vi "PC_AIChar.vi"() -> ()   [LabVIEW 2017]
uses:
  <vilib>/NI/STM/NI STM.lvlib
  <vilib>/Analysis/NI_AALBase.lvlib
  <vilib>/measure/NI_MAPro.lvlib
  <vilib>/measure/maspectr.llb/Power Spectrum and PSD Export Mode.ctl
  <vilib>/Analysis/NI_AALPro.lvlib
  Components/TypeDefs/UIStateDefEnum.ctl
  Components/Spectra/Spectra.lvlib
  <vilib>/NI/STM/TCP/Read Message (TCP).vi
  <vilib>/Analysis/5stat.llb/RMS (DBL).vi
  <vilib>/measure/maspectr.llb/FFT Power Spectrum and PSD for 1 Chan.vi
  <vilib>/Analysis/baseanly.llb/Mean (DBL).vi
  <vilib>/NI/STM/TCP/Read Meta Data (TCP Ref).vi
  <vilib>/NI/STM/TCP/Get Connection Reference (TCP).vi
panel:
  out "Analysis Loop \ntime [s]":dbl format="%#.4g"
  out "Analysis \ntime-span [s]":dbl format="%.2f"
  out "# of elements \nremoved":i32
  in  "Pause Charts":bool
  in  "Clear charts":bool
  out "RT target \nloop \ntime [s]":dbl=0.0002
  out "Data length \n[count]":i32
  out "Mean [V]":dbl format="%#.6f"
  out "RMS / \nStd. Dev. [mV]":dbl format="%#.6f"
  out "Spectra plots":cluster{"f0":dbl, "df":dbl, "magnitude":dbl[]}[](graph)
  out "Histogram Graph":T1(graph)
  out "STM Loop \ntime [s]":dbl format="%#.4g"
  in  "System Stop Button":bool
  out "Data":dbl[][](graph)
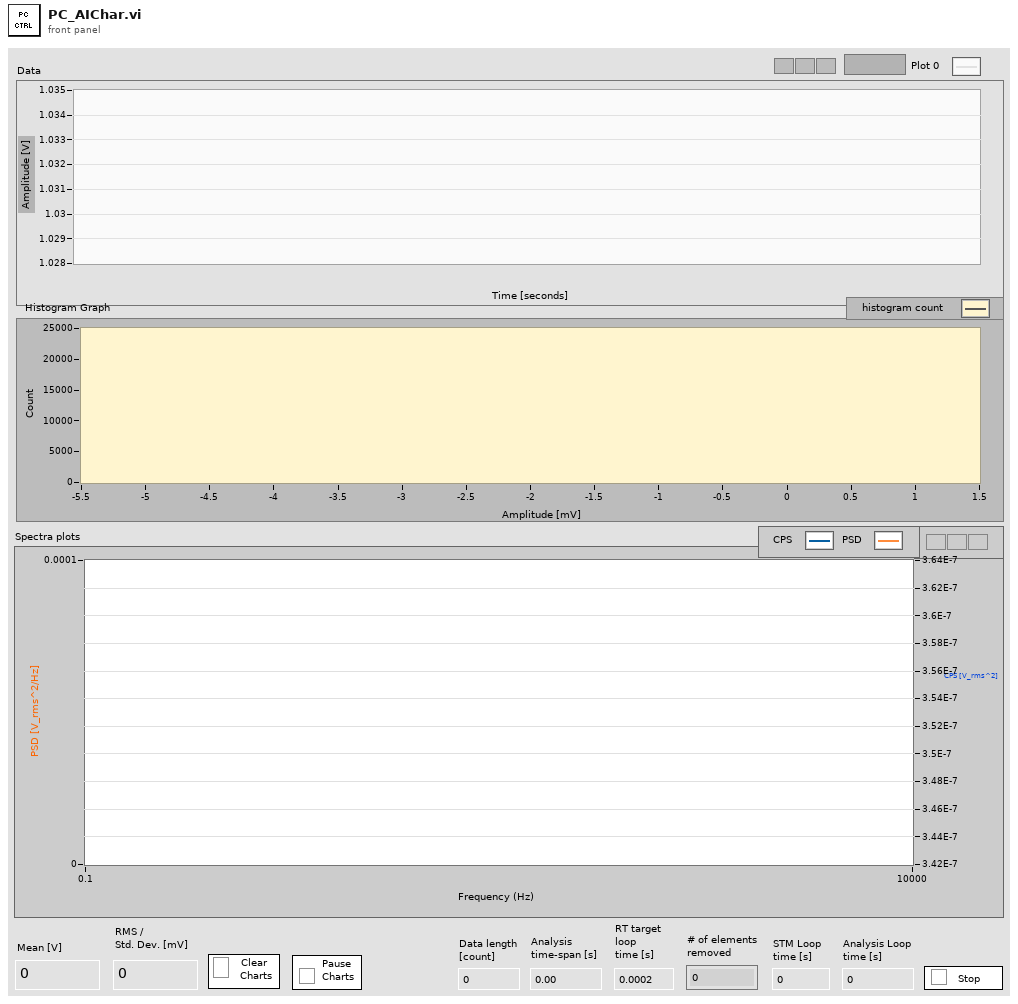
[diagram p1: front panel]
types:
  T1 = cluster{"X Values":dbl[], "Histogram: h(x)":i32[]}
  T2 = typedef "UIStateDefEnum.ctl" = enum16{"Wait", "Initialize", "Clear", "Stop"}
  T3 = typedef "NI STM.lvlib/TCP Connection Info.ctl" = cluster{"connection ID":refnum<k5>, "meta data":T4[]}
  T4 = typedef "NI STM.lvlib/MetaDataElement.ctl" = string
  T5 = typedef "NI_MAPro.lvlib/Power Spectrum and PSD Export Mode.ctl" = u16
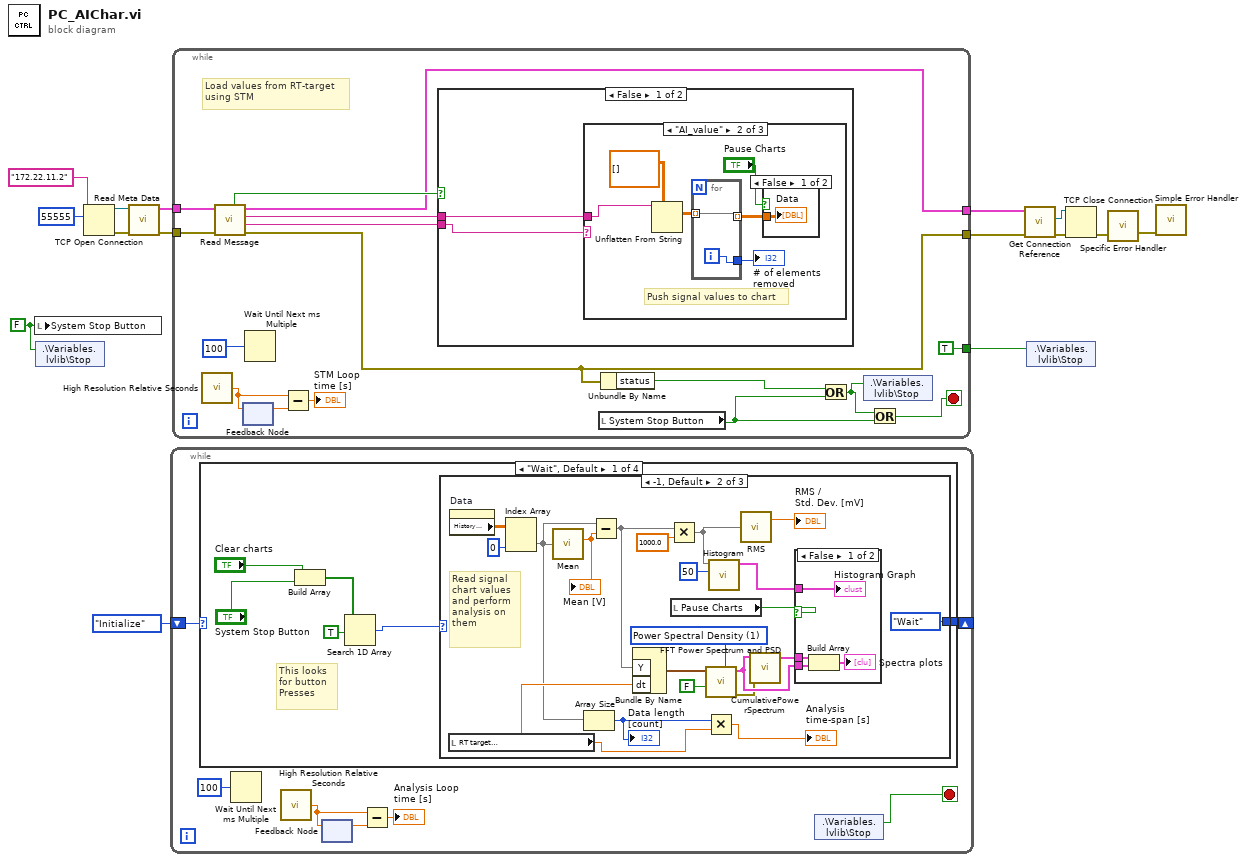
[diagram p0: block diagram]
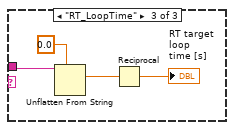
[diagram p4: hidden frame]
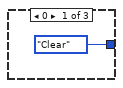
[diagram p6: hidden frame]
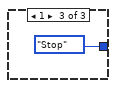
[diagram p8: hidden frame]
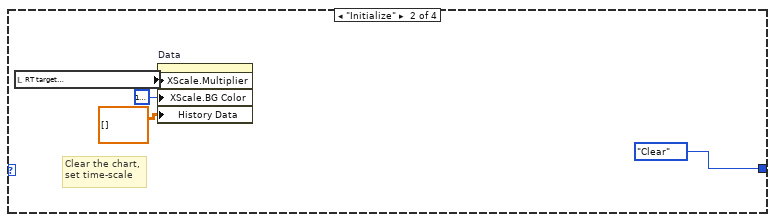
[diagram p9: hidden frame]
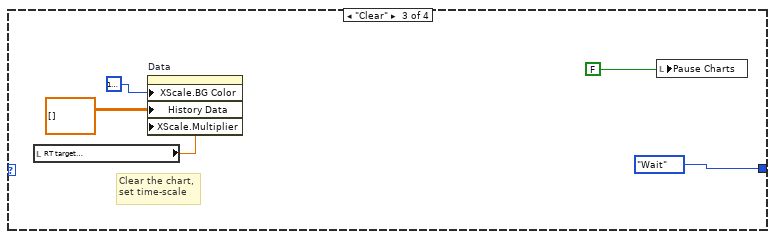
[diagram p10: hidden frame]
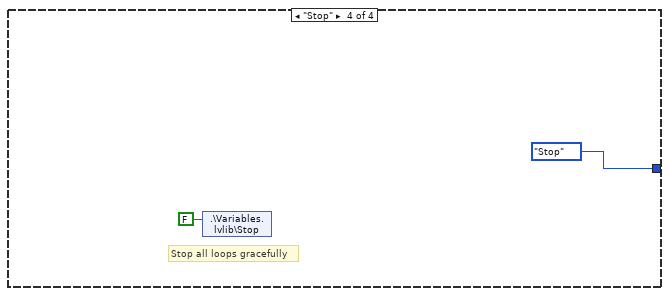
[diagram p11: hidden frame]
diagram:
  w3 = FALSE ("System Stop Button")
  n1 = local write "System Stop Button"(w3) -> ()
  n2 = shared-variable ".\\Variables.lvlib\\Stop"(w3) -> ()  [unwired: 1 in, 1 out]
  n3 = TCP Open Connection(address="172.22.11.2", remote port or service name=u16 55555) -> (connection ID=w13:refnum<k5>, error out=w12:errorcluster)  [unwired: 3 in]
  n4 = call-poly <vilib>:"Read Meta Data.vi"("error in"=w12, "connection ID"=w13) -> ("error out"=w10:errorcluster, "connection info out"=w11:T3)  [unwired: 7 in, 1 out]
  n5 = while {
    shift-right: [w20] -> _
    shift-left: UIStateDefEnum."Initialize" ("UIStateDefEnum") -> [w21]
    stop <- w19 stop-if-true
    n6 = case shown="\"Wait\", Default" w21 {
      tunnel: [w23 UIStateDefEnum."Clear" ("UIStateDefEnum") UIStateDefEnum."Wait" ("UIStateDefEnum") UIStateDefEnum."Stop" ("UIStateDefEnum")] -> w20
      frame "Wait", Default {
        # "This looks \nfor button \nPresses"
        n7 = Build Array "Build Array"("Clear charts", "System Stop Button") -> (w28:bool[])
        n8 = Search 1D Array(1D array=w28, element=TRUE) -> (index of element=w24:i32)  [unwired: 1 in]
        n9 = case shown="-1, Default" w24 {
          tunnel: [UIStateDefEnum."Clear" ("UIStateDefEnum") UIStateDefEnum."Wait" ("UIStateDefEnum") UIStateDefEnum."Stop" ("UIStateDefEnum")] -> w23
          frame 0 {
          }
          frame -1, Default {
            w46 = T5 1 items=["Power Spectrum", "Power Spectral Density"] ("export mode")
            # "Read signal\nchart values\nand perform\nanalysis on \nthem"
            n10 = local read "RT target \nloop \ntime [s]"() -> (w39:dbl)
            n11 = property on="Data" class="WFChart (strict)"() -> ("History Data"=w44:dbl[][])  [unwired: 2 in, 2 out]
            n12 = Index Array(array=w44, index (col)=0 ("disabled index (col)")) -> (element=w34:dbl[])  [unwired: 1 in]
            n13 = call-poly <vilib>:"Mean.vi"("X"=w34) -> ("mean"=w45:dbl)  [unwired: 1 out]
            "Mean [V]" <- w45
            n14 = Array Size(array=w34) -> (size(s)=w40:i32)
            "Data length \n[count]" <- w40
            n15 = Subtract(x=w34, y=w45) -> (x-y=w33:dbl[])
            n16 = Bundle By Name("Y"=w33, "dt"=w39) -> (w48:waveform(dbl))  [unwired: 1 in]
            n17 = Multiply(x=w33, y=1000.0) -> (x*y=w35:dbl[])
            n18 = local read "Pause Charts"() -> (w38:bool)
            n19 = call-poly <vilib>:"FFT Power Spectrum and PSD.vi"("export mode"=w46, "dB On (F)"=FALSE, "time signal"=w48) -> ("error out"=w30:errorcluster, "Power Spectrum / PSD"=w31:cluster{"f0":dbl, "df":dbl, "magnitude":dbl[]})  [unwired: 5 in, 2 out]
            n20 = Multiply(x=w40, y=w39) -> (x*y=→"Analysis \ntime-span [s]":dbl)
            n21 = call <vilib>:"Histogram.vi"("intervals"=50, "X"=w35) -> ("Histogram Graph"=w49:T1)  [unwired: 6 in, 3 out]
            n22 = call-poly <vilib>:"RMS.vi"("X"=w35) -> ("rms value"=→"RMS / \nStd. Dev. [mV]":dbl)  [unwired: 1 out]
            n23 = call "CumulativePowerSpectrum.vi"("error in (no error)"=w30, "PSD"=w31) -> ("CPS"=w32:cluster{"f0":dbl, "df":dbl, "magnitude":dbl[]})  [unwired: 8 in, 1 out]
            n24 = case shown="False" w38 {
              tunnel: w49 -> [w54 _]
              tunnel: w32 -> [w53 _]
              tunnel: w31 -> [w51 _]
              frame False {
                n25 = Build Array(w53, w51) -> (→"Spectra plots":cluster{"f0":dbl, "df":dbl, "magnitude":dbl[]}[])
                "Histogram Graph" <- w54
              }
              frame True {
              }
            }
          }
          frame 1 {
          }
        }
      }
      frame "Initialize" {
        # "Clear the chart,\nset time-scale"
        n26 = local read "RT target \nloop \ntime [s]"() -> (w58:dbl)
        n27 = property on="Data" class="WFChart (strict)"("XScale.Multiplier"=w58, "XScale.BG Color"=u32 16777216 ("X Scale.Marker Colors:BG Color"), "History Data"=dbl[][] []) -> ()  [unwired: 2 in, 2 out]
      }
      frame "Clear" {
        # "Clear the chart,\nset time-scale"
        n28 = local read "RT target \nloop \ntime [s]"() -> (w60:dbl)
        n29 = property on="Data" class="WFChart (strict)"("XScale.BG Color"=u32 16777216 ("X Scale.Marker Colors:BG Color"), "History Data"=dbl[][] [], "XScale.Multiplier"=w60) -> ()  [unwired: 2 in, 2 out]
        n30 = local write "Pause Charts"(FALSE ("Pause Charts")) -> ()
      }
      frame "Stop" {
        # "Stop all loops gracefully"
        n31 = shared-variable ".\\Variables.lvlib\\Stop"(FALSE ("Stop")) -> ()  [unwired: 1 in, 1 out]
      }
    }
    n32 = Wait Until Next ms Multiple(millisecond multiple=u32 100) -> ()  [unwired: 1 out]
    n33 = call <vilib>:"High Resolution Relative Seconds.vi"() -> ("relative seconds"=w17:dbl)
    n34 = feedback #1() -> (w18:dbl)  [unwired: 1 in]
    n35 = feedback-in #1(w17) -> ()
    n36 = Subtract(x=w17, y=w18) -> (x-y=→"Analysis Loop \ntime [s]":dbl)
    n37 = shared-variable ".\\Variables.lvlib\\Stop"() -> (w19:bool)  [unwired: 1 in, 1 out]
  }
  n38 = while {
    tunnel: w11 -> [w82]
    tunnel: w10 -> [w81]
    tunnel: [w79] -> w6
    tunnel: [w78] -> w5
    tunnel: [TRUE ("Stop")] -> w1
    stop <- w72 stop-if-true
    # "Load values from RT-target\nusing STM"
    n39 = call <vilib>:"High Resolution Relative Seconds.vi"() -> ("relative seconds"=w74:dbl)
    n40 = call-poly <vilib>:"Read Message.vi"("error in"=w81, "connection info in"=w82) -> ("error out"=w78:errorcluster, "name"=w77:T4, "data string"=w76:string, "connection info out"=w79:T3, "timed out?"=w80:bool)  [unwired: 4 in, 1 out]
    n41 = feedback-in #2(w74) -> ()
    n42 = feedback #2() -> (w75:dbl)  [unwired: 1 in]
    n43 = Wait Until Next ms Multiple(millisecond multiple=u32 100 ("Period")) -> ()  [unwired: 1 out]
    n44 = Subtract(x=w74, y=w75) -> (x-y=→"STM Loop \ntime [s]":dbl)
    n45 = case shown="False" w80 {
      tunnel: w77 -> [w84 _]
      tunnel: w76 -> [w83 _]
      frame False {
        n46 = case shown="\"AI_value\"" w84 {
          tunnel: w83 -> [_ w89 w94]
          frame Default {
          }
          frame "AI_value" {
            # "Push signal values to chart"
            n47 = Unflatten From String(type=dbl[][] [], binary string=w89) -> (value=w88:dbl[][])  [unwired: 3 in, 2 out]
            n48 = for {
              tunnel: w88 -> [w93] mode=indexing
              tunnel: [w93] -> w87 mode=indexing
              tunnel: [w92] -> w86
              i -> [w92]
            }
            "# of elements \nremoved" <- w86
            n49 = case shown="False" "Pause Charts" {
              tunnel: w87 -> [w91 _]
              frame False {
                "Data" <- w91
              }
              frame True {
              }
            }
          }
          frame "RT_LoopTime" {
            n50 = Unflatten From String(type=0.0, binary string=w94) -> (value=w96:dbl)  [unwired: 3 in, 2 out]
            n51 = Reciprocal(x=w96) -> (1/x=→"RT target \nloop \ntime [s]":dbl)
          }
        }
      }
      frame True {
      }
    }
    n52 = local read "System Stop Button"() -> (w71:bool)
    n53 = Unbundle By Name(w78) -> ("status"=w70:bool)
    n54 = Or(x=w70, y=w71) -> (x .or. y?=w69:bool)
    n55 = shared-variable ".\\Variables.lvlib\\Stop"(w69) -> ()  [unwired: 1 in, 1 out]
    n56 = Or(x=w69, y=w71) -> (x .or. y?=w72:bool)
  }
  n57 = call-poly <vilib>:"Get Connection Reference.vi"("error in"=w5, "connection info in"=w6) -> ("error out"=w9:errorcluster, "connection ID out"=w8:refnum<k5>)  [unwired: 7 in, 1 out]
  n58 = shared-variable ".\\Variables.lvlib\\Stop"(w1) -> ()  [unwired: 1 in, 1 out]
  n59 = TCP Close Connection(connection ID=w8, error in (no error)=w9) -> (error out=w7:errorcluster)  [unwired: 1 in, 1 out]
  n60 = call "Specific Error Handler"("Error to Check"=w7) -> ("error out"=w4:errorcluster)  [unwired: 11 in, 3 out]
  n61 = call <vilib>:"Simple Error Handler.vi"("error in (no error)"=w4) -> ()  [unwired: 4 in, 5 out]
